vi "Create Dataset 1D Double.vi"(7 "Chunk size":u64, 8 "error in (no error)":errorcluster, 9 "Datatype":i32[](array[numeric]), 10 "Dataset name":string, 11 "Location id in":i32) -> (0 "error out":errorcluster, 3 "dataset_id":i32)   [LabVIEW 2016]
uses:
  Release/HDF5Tools.dll
  HDF5Tools.lvlib
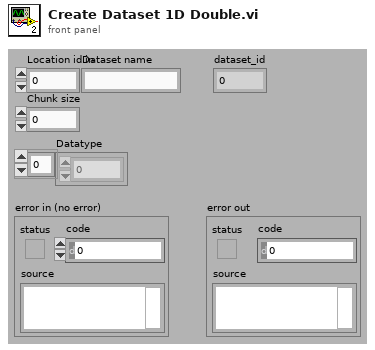
[diagram p1: front panel]
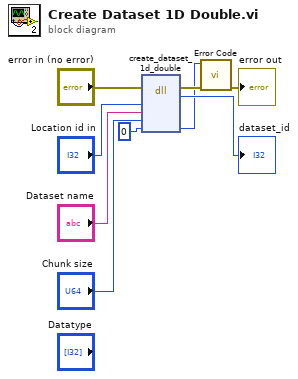
[diagram p0: block diagram]
diagram:
  n1 = dll-call lib="Z:/users/Manolis/Labview/Cajal/private/HDF5Tools32/Release/HDF5Tools.dll" fn="create_dataset_1d_double"(error in="error in (no error)", "loc_id"="Location id in", "name"="Dataset name", "chunk"="Chunk size", "error"=0) -> (error out=w4:errorcluster, "dataset_id"=→"dataset_id":i32, "error"=w2:i32)  [unwired: 5 in, 1 out]
  n2 = call "Error Code.vi"("Error in"=w4, "Error code"=w2) -> ("Error out"=→"error out":errorcluster)  [unwired: 9 in]
